vi "SortFileNames.vi"(6 "Tags":T1={"Pattern (eg. H,V)"="H,V", "File type"={"AvR"=TRUE, "AvC"=FALSE, "trf"=FALSE, "wfm"=FALSE, "All"=FALSE}, "keywords 1"="", "keywords 2"="", "keywords 3"=""}, 10 "Listing Order":T2(ring), 11 "Files in":path[](array[path])) -> (1 "wfm only?":bool, 3 "Files out":path[](array[path]))   [LabVIEW 2022 SP3]
panel:
  out "sorted":dbl[](array[numeric])
  # "Or"
  # "Or"
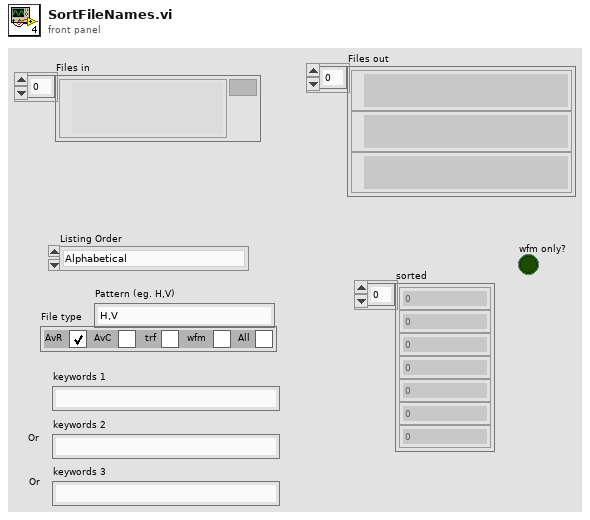
[diagram p1: front panel]
types:
  T1 = cluster{"Pattern (eg. H,V)":string, "File type":cluster{"AvR":bool, "AvC":bool, "trf":bool, "wfm":bool, "All":bool}, "keywords 1":string, "keywords 2":string, "keywords 3":string}
  T2 = enum16{"Alphabetical", "Chronological", "Hit Strength (min to max)", "Hit Strength (max to min)"}
  T3 = cluster{"AvR":bool, "AvC":bool, "trf":bool, "wfm":bool, "All":bool}
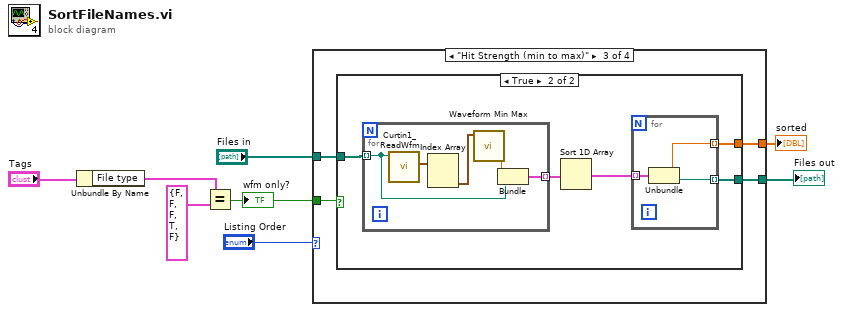
[diagram p0: block diagram]
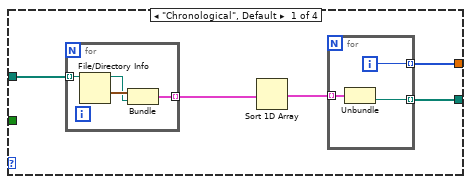
[diagram p2: hidden frame]
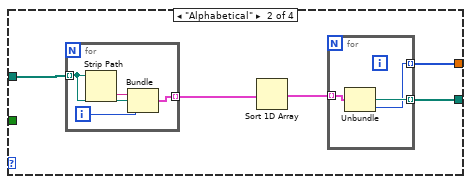
[diagram p3: hidden frame]
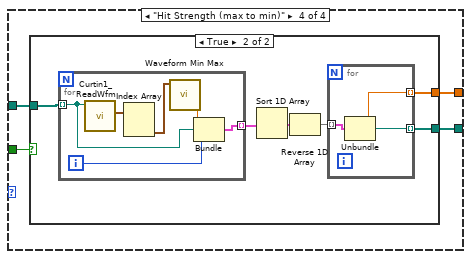
[diagram p5: hidden frame]
diagram:
  n1 = Unbundle By Name("Tags") -> ("File type"=w2:T3)
  n2 = Equal?(x=w2, y=T3 {"AvR"=FALSE, "AvC"=FALSE, "trf"=FALSE, "wfm"=TRUE, "All"=FALSE} ("File type")) -> (x = y?=w1:bool)
  "wfm only?" <- w1
  n3 = case shown="\"Hit Strength (min to max)\"" "Listing Order" {
    tunnel: "Files in" -> [w13 w25 w36 w54]
    tunnel: [w10 w22 w35 w53] -> w6
    tunnel: [w9 w21 w34 w52] -> w5
    tunnel: w1 -> [_ _ w33 w51]
    frame "Chronological", Default {
      n4 = for {
        tunnel: w13 -> [w20] mode=indexing
        tunnel: [w17] -> w12 mode=indexing
        n5 = File/Directory Info(path=w20) -> (path out=w18:path, last mod=w19:timestamp)  [unwired: 1 in, 5 out]
        n6 = Bundle("last mod"=w19, "path out"=w18) -> (w17:cluster{"last mod":timestamp, "path out":path})  [unwired: 1 in]
      }
      n7 = Sort 1D Array(array=w12) -> (sorted array=w11:cluster{"last mod":timestamp, "path out":path}[])
      n8 = for {
        tunnel: w11 -> [w16] mode=indexing
        tunnel: [w15] -> w10 mode=indexing
        tunnel: [w14] -> w9 mode=indexing
        i -> [w14]
        n9 = Unbundle(w16) -> ("path out"=w15:path)  [unwired: 1 out]
      }
    }
    frame "Alphabetical" {
      n10 = for {
        tunnel: w25 -> [w29] mode=indexing
        tunnel: [w32] -> w24 mode=indexing
        i -> [w30]
        n11 = Strip Path(path=w29) -> (name=w31:string)  [unwired: 1 out]
        n12 = Bundle("name"=w31, "Path out"=w29, w30) -> (w32:cluster{"name":string, "Path out":path, i32})  [unwired: 1 in]
      }
      n13 = Sort 1D Array(array=w24) -> (sorted array=w23:cluster{"name":string, "Path out":path, i32}[])
      n14 = for {
        tunnel: w23 -> [w28] mode=indexing
        tunnel: [w27] -> w22 mode=indexing
        tunnel: [w26] -> w21 mode=indexing
        n15 = Unbundle(w28) -> ("Path out"=w27:path, w26:i32)  [unwired: 1 out]
      }
    }
    frame "Hit Strength (min to max)" {
      n16 = case shown="True" w33 {
        tunnel: w36 -> [w37 w42]
        tunnel: [w37 w39] -> w35
        tunnel: [_ w38] -> w34
        frame False {
        }
        frame True {
          n17 = for {
            tunnel: w42 -> [w46] mode=indexing
            tunnel: [w50] -> w41 mode=indexing
            n18 = call "Curtin1_ReadWfm.vi"("appended path"=w46) -> ("all waveforms in record"=w49:waveform(dbl)[])  [unwired: 9 in, 1 out]
            n19 = Index Array(array=w49) -> (element #2=w48:waveform(dbl))  [unwired: 2 in, 1 out]
            n20 = call <vilib>:"Waveform Min Max.vi"("waveform in"=w48) -> ("Y max"=w47:dbl)  [unwired: 5 in, 5 out]
            n21 = Bundle("Y max"=w47, "Path out"=w46) -> (w50:cluster{"Y max":dbl, "Path out":path})  [unwired: 1 in]
          }
          n22 = Sort 1D Array(array=w41) -> (sorted array=w40:cluster{"Y max":dbl, "Path out":path}[])
          n23 = for {
            tunnel: w40 -> [w45] mode=indexing
            tunnel: [w44] -> w39 mode=indexing
            tunnel: [w43] -> w38 mode=indexing
            n24 = Unbundle(w45) -> ("Y max"=w43:dbl, "Path out"=w44:path)
          }
        }
      }
    }
    frame "Hit Strength (max to min)" {
      n25 = case shown="True" w51 {
        tunnel: w54 -> [w55 w61]
        tunnel: [w55 w58] -> w53
        tunnel: [_ w57] -> w52
        frame False {
        }
        frame True {
          n26 = for {
            tunnel: w61 -> [w66] mode=indexing
            tunnel: [w70] -> w60 mode=indexing
            i -> [w65]
            n27 = call "Curtin1_ReadWfm.vi"("appended path"=w66) -> ("all waveforms in record"=w69:waveform(dbl)[])  [unwired: 9 in, 1 out]
            n28 = Index Array(array=w69) -> (element #2=w68:waveform(dbl))  [unwired: 2 in, 1 out]
            n29 = call <vilib>:"Waveform Min Max.vi"("waveform in"=w68) -> ("Y max"=w67:dbl)  [unwired: 5 in, 5 out]
            n30 = Bundle("Y max"=w67, "Path out"=w66, w65) -> (w70:cluster{"Y max":dbl, "Path out":path, i32})  [unwired: 1 in]
          }
          n31 = Sort 1D Array(array=w60) -> (sorted array=w59:cluster{"Y max":dbl, "Path out":path, i32}[])
          n32 = Reverse 1D Array(array=w59) -> (reversed array=w56:cluster{"Y max":dbl, "Path out":path, i32}[])
          n33 = for {
            tunnel: w56 -> [w64] mode=indexing
            tunnel: [w63] -> w58 mode=indexing
            tunnel: [w62] -> w57 mode=indexing
            n34 = Unbundle(w64) -> ("Y max"=w62:dbl, "Path out"=w63:path)  [unwired: 1 out]
          }
        }
      }
    }
  }
  "Files out" <- w6
  "sorted" <- w5
